vi "find_optimal_control_parameters.vi"() -> ()   [LabVIEW 2017]
uses:
  <vilib>/DAQmx/write.llb/DAQmx Write (Analog 1D Wfm NChan NSamp).vi
  <vilib>/DAQmx/create/channels.llb/DAQmx Create Channel (AO-Voltage-Basic).vi
  <vilib>/DAQmx/configure/timing.llb/DAQmx Timing (Sample Clock).vi
  <vilib>/DAQmx/miscellaneous.llb/DAQmx Fill In Error Info.vi
panel:
  in  "Camera delay (s)":dbl=0.5
  in  "Camera start phase":dbl=63.0
  in  "Exposure Time":dbl=0.00199
  in  "Camera Region":T1={"Horizontal Offset"=1020, "Vertical Offset"=820, "Horizontal Size"=580, "Vertical Size"=404}
  out "XY Graph":cluster{"Array":dbl[], "Array":dbl[]}(graph)
  in  "Stop":bool
  out "error out":errorcluster
  in  "Save data path":path=path "D:/"
  in  "Project name":string="syn data"
  in  "Number of Samples":i32=400000
  in  "Sample Rate":dbl=400000.0
  in  "Sample Clock Source":tag="OnboardClock"
  in  "Max Voltage":dbl=5.0
  in  "Min Voltage":dbl=-1.0
  in  "Physical Channel(s)":tag="PXI1Slot3_2/ao29, PXI1Slot3_2/ao31, PXI1Slot3_2/ao3"
  in  "Tab Control":T2(tab)
  in  "Frequency":dbl=50.0
  in  "Vgalvo phase Max":dbl=123.0
  in  "Vgalvo phase Min":dbl=113.0
  out "Vgalvo phase":dbl
  in  "Vgalvo offset":dbl
  in  "Vgalvo amplitude":dbl=0.068
  in  "Iteration times":i32=10
  in  "Vetl phase":dbl
  in  "Vetl amplitude":dbl=0.8
  in  "Vetl offset":dbl=2.0
  out "Vgalvo offset 2":dbl
  in  "Vgalvo offset Max 2":dbl=0.01
  in  "Vgalvo offset Min 2":dbl=-0.01
  in  "Iteration times 2":i32=10
  in  "Vgalvo phase 2":dbl=118.0
  in  "Vgalvo amplitude 2":dbl=0.068
  in  "Vetl phase 2":dbl
  in  "Vetl amplitude 2":dbl=0.8
  in  "Vetl offset 2":dbl=2.0
  in  "Frequency 2":dbl=50.0
  out "Vgalvo amp 3":dbl
  in  "Vgalvo amp Max 3":dbl=0.07
  in  "Vgalvo amp Min 3":dbl=0.066
  in  "Iteration times 3":i32=10
  in  "Vgalvo phase 3":dbl=118.0
  in  "Vgalvo offset 3":dbl
  in  "Vetl phase 3":dbl
  in  "Vetl amplitude 3":dbl=0.8
  in  "Vetl offset 3":dbl=2.0
  in  "Frequency 3":dbl=50.0
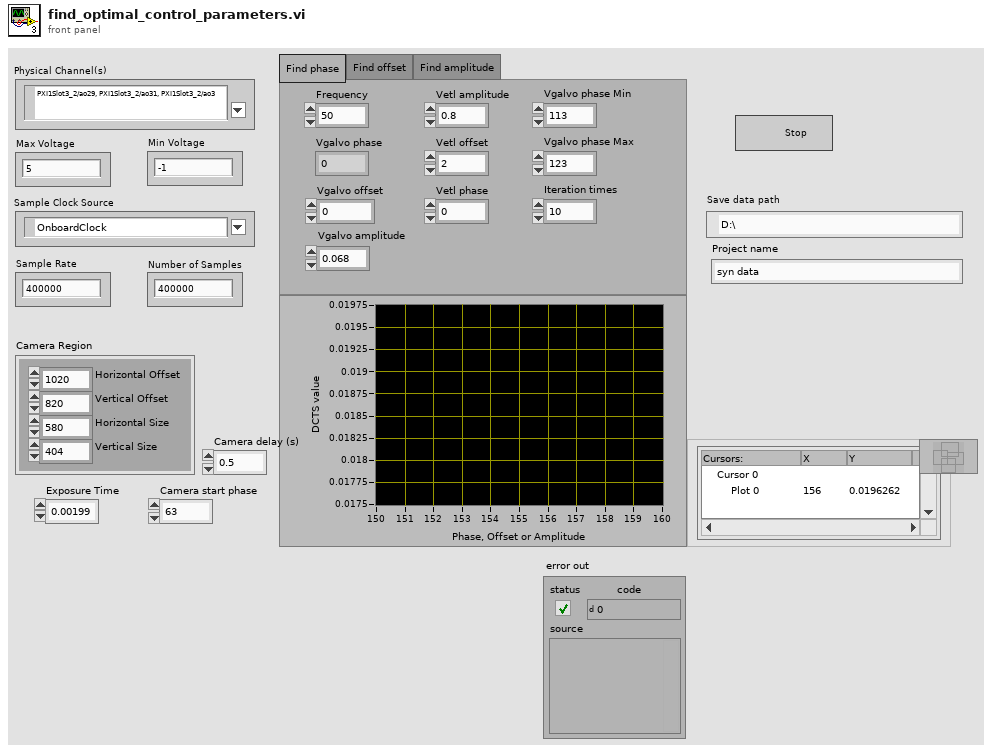
[diagram p1: front panel]
types:
  T1 = cluster{"Horizontal Offset":i32, "Vertical Offset":i32, "Horizontal Size":i32, "Vertical Size":i32}
  T2 = enum32{"Find phase", "Find offset", "Find amplitude"}
  T3 = enum16{"open", "replace", "create", "open or create", "replace or create", "replace or create with confirmation"}
  T4 = cluster{"frequency":dbl, "amplitude":dbl, "offset":dbl, "phase":dbl}
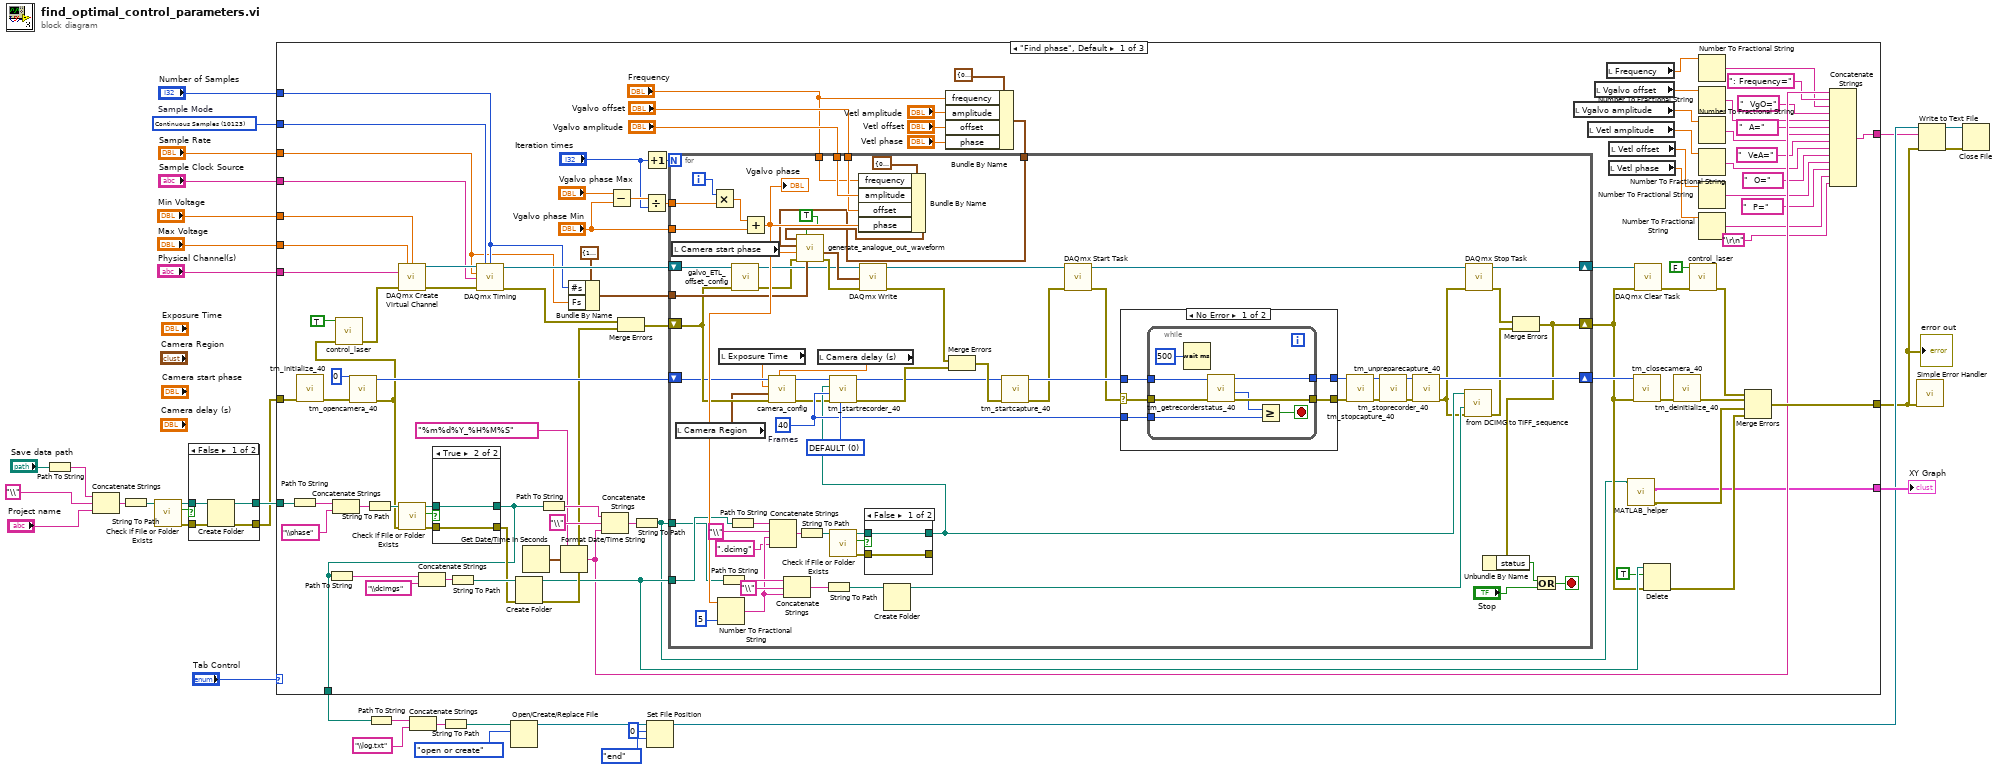
[diagram p0: block diagram]
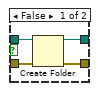
[diagram p3: hidden frame]
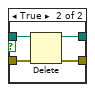
[diagram p5: hidden frame]
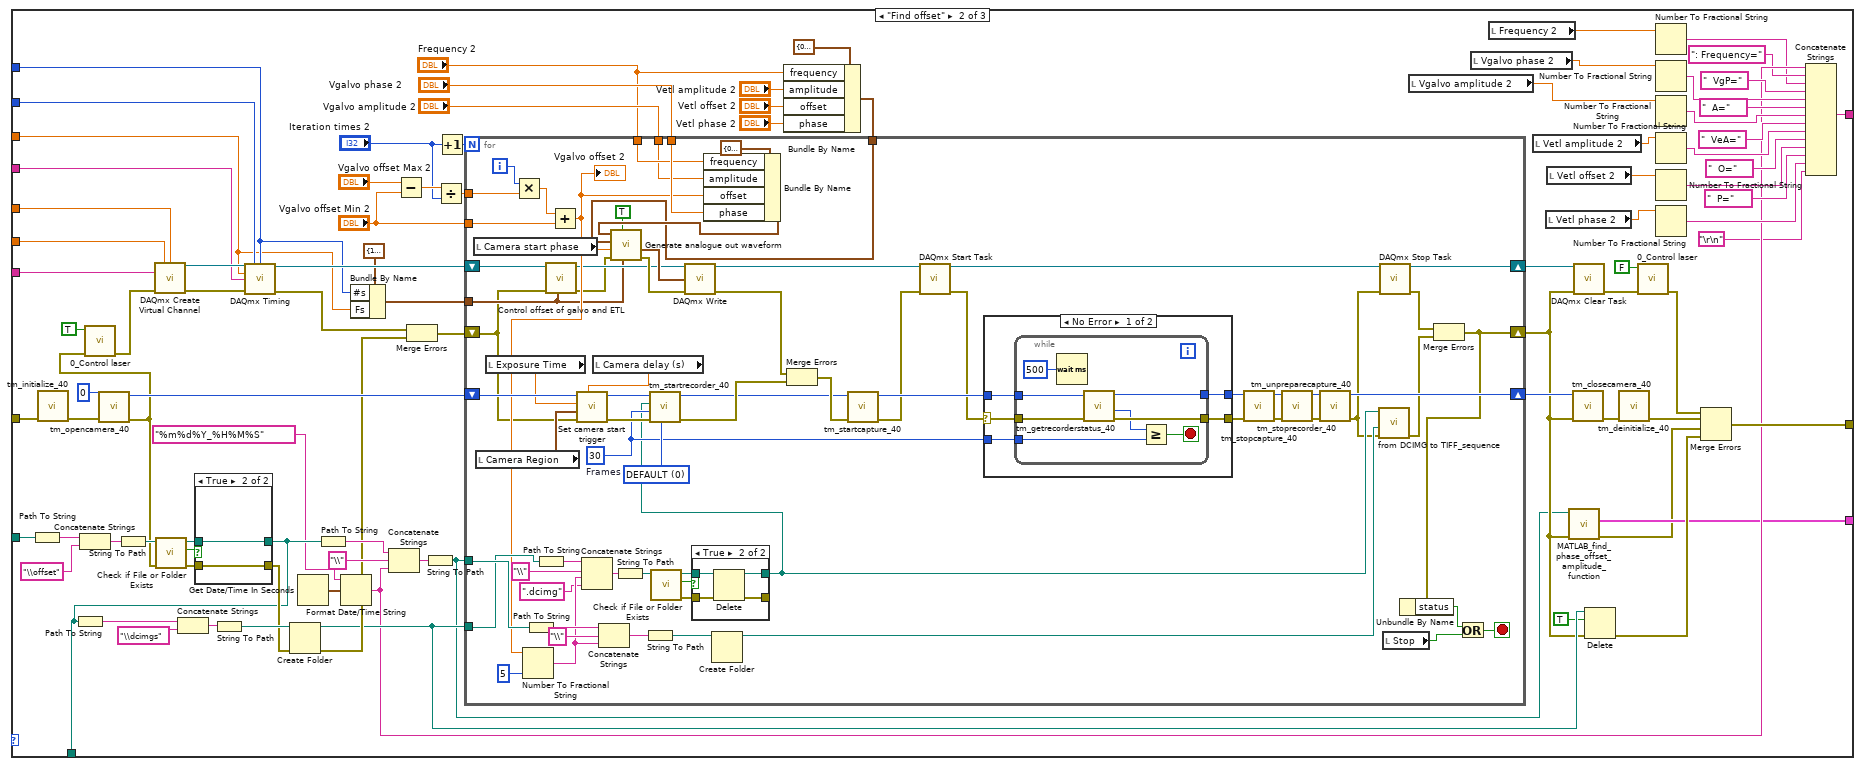
[diagram p6: hidden frame]
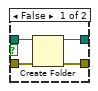
[diagram p7: hidden frame]
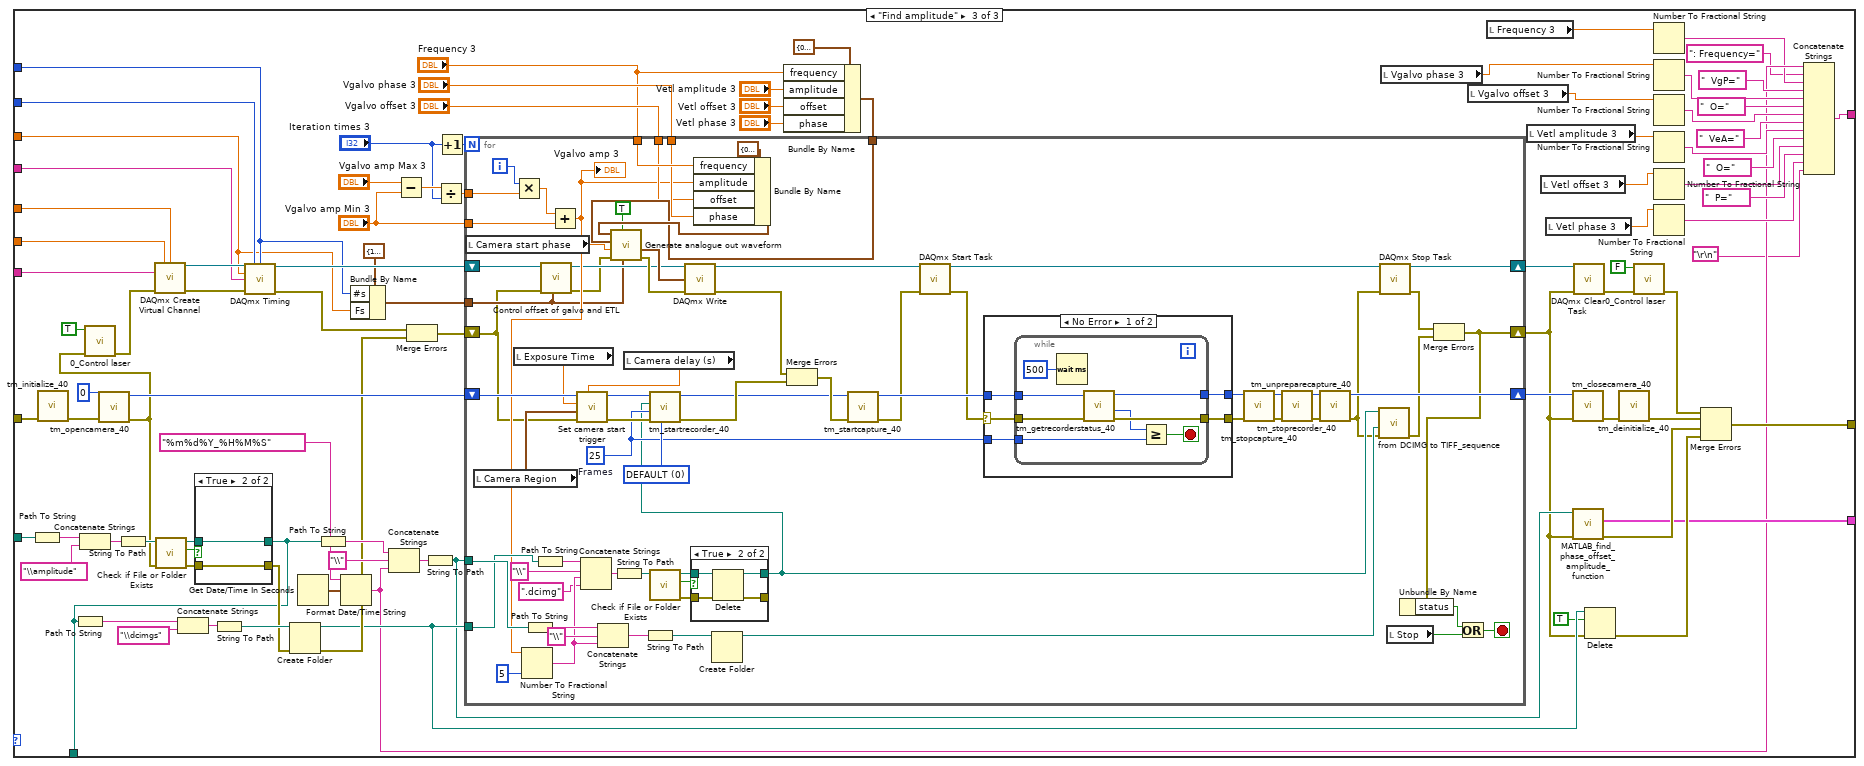
[diagram p10: hidden frame]
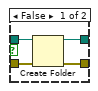
[diagram p11: hidden frame]
diagram:
  w23 = 10123 items=["Finite Samples"=10178, "Continuous Samples"=10123, "Hardware Timed Single Point"=12522]  # Sample Mode
  n1 = Path To String(path="Save data path") -> (string=w28:string)
  n2 = Concatenate Strings(w28, "\\", "Project name") -> (w27:string)
  n3 = String To Path(string=w27) -> (path=w33:path)
  n4 = call <vilib>:"Check if File or Folder Exists.vi"("path"=w33) -> ("error out"=w32:errorcluster, "file or folder exists?"=w31:bool, "dup path"=w30:path)  [unwired: 8 in]
  n5 = case shown="False" w31 {
    tunnel: w30 -> [w38 w39]
    tunnel: w32 -> [w37 w40]
    tunnel: [w36 w40] -> w1
    tunnel: [w35 w39] -> w26
    frame False {
      n6 = Create Folder(path (use dialog)=w38, error in=w37) -> (created path=w35:path, error out=w36:errorcluster)  [unwired: 1 in, 1 out]
    }
    frame True {
    }
  }
  n7 = case shown="\"Find phase\", Default" "Tab Control" {
    tunnel: w26 -> [w128 w264 w448]
    tunnel: w1 -> [w108 w263 w449]
    tunnel: w23 -> [w90 w270 w455]
    tunnel: "Number of Samples" -> [w84 w271 w456]
    tunnel: "Sample Rate" -> [w83 w269 w454]
    tunnel: "Sample Clock Source" -> [w89 w268 w453]
    tunnel: "Min Voltage" -> [w88 w267 w452]
    tunnel: "Max Voltage" -> [w87 w266 w451]
    tunnel: "Physical Channel(s)" -> [w86 w265 w450]
    tunnel: [w73 w262 w446] -> w3
    tunnel: [w44 w238 w447] -> w16
    tunnel: [w71 w250 w434] -> w12
    tunnel: [w53 w251 w435] -> w5
    frame "Find phase", Default {
      n8 = Path To String(path=w128) -> (string=w127:string)
      n9 = call <userlib>:"tm_initialize_40.vi"("error in (no error)"=w108) -> ("error out"=w123:errorcluster)  [unwired: 7 in, 3 out]
      n10 = Concatenate Strings(w127, "\\phase") -> (w125:string)
      n11 = call <userlib>:"tm_opencamera_40.vi"("error in (no error)"=w123, "Camera Index"=u32 0) -> ("error out"=w48:errorcluster, "Handle out"=w117:u32)  [unwired: 7 in, 1 out]
      n12 = call "control_laser.vi"("error in (no error)"=w48, "Laser On/Off"=TRUE ("Layser On/Off")) -> ("error out"=w49:errorcluster)  [unwired: 9 in]
      n13 = String To Path(string=w125) -> (path=w124:path)
      n14 = call-poly <vilib>:"DAQmx Create Virtual Channel.vi"("maximum value"=w87, "minimum value"=w88, "physical channels"=w86, "error in"=w49) -> ("task out"=w110:refnum<k21>, "error out"=w109:errorcluster)  [unwired: 10 in]
      n15 = call <vilib>:"Check if File or Folder Exists.vi"("error in (no error)"=w48, "path"=w124) -> ("error out"=w131:errorcluster, "file or folder exists?"=w130:bool, "dup path"=w129:path)  [unwired: 7 in]
      n16 = case shown="True" w130 {
        tunnel: w129 -> [w135 w136]
        tunnel: w131 -> [w134 w137]
        tunnel: [w133 w137] -> w93
        tunnel: [w132 w136] -> w71
        frame False {
          n17 = Create Folder(path (use dialog)=w135, error in=w134) -> (created path=w132:path, error out=w133:errorcluster)  [unwired: 1 in, 1 out]
        }
        frame True {
        }
      }
      n18 = Path To String(path=w71) -> (string=w118:string)
      n19 = Concatenate Strings(w118, "\\dcimgs") -> (w120:string)
      n20 = String To Path(string=w120) -> (path=w119:path)
      n21 = call-poly <vilib>:"DAQmx Timing.vi"("task/channels in"=w110, "sample mode"=w90, "samples per channel"=w84, "rate"=w83, "source"=w89, "error in"=w109) -> ("task out"=w105:refnum<k21>, "error out"=w94:errorcluster)  [unwired: 8 in]
      n22 = Create Folder(path (use dialog)=w119, error in=w93) -> (created path=w78:path, error out=w92:errorcluster)  [unwired: 1 in, 1 out]
      n23 = Get Date/Time In Seconds() -> (seconds since 1Jan1904=w104:timestamp)
      n24 = Path To String(path=w71) -> (string=w101:string)
      n25 = Format Date/Time String(time format string (%c)="%m%d%Y_%H%M%S", seconds (now)=w104) -> (date/time string=w64:string)  [unwired: 1 in]
      n26 = Bundle By Name(cluster=cluster{"Fs":dbl, "#s":dbl} {"Fs"=1000.0, "#s"=1000.0} ("sampling info"), "#s"=w84, "Fs"=w83) -> (w82:cluster{"Fs":dbl, "#s":dbl})
      n27 = Concatenate Strings(w101, "\\", w64) -> (w102:string)
      n28 = Subtract(x="Vgalvo phase Max", y="Vgalvo phase Min") -> (x-y=w115:dbl)
      n29 = Merge Errors(w94, w92) -> (w91:errorcluster)
      n30 = String To Path(string=w102) -> (path=w45:path)
      n31 = Divide(x=w115, y="Iteration times") -> (x/y=w112:dbl)
      n32 = Increment(x="Iteration times") -> (x+1=w113:i32)
      n33 = Bundle By Name(cluster=T4 {"frequency"=0.0, "amplitude"=0.0, "offset"=0.0, "phase"=0.0}, "frequency"="Frequency", "amplitude"="Vetl amplitude", "offset"="Vetl offset", "phase"="Vetl phase") -> (w95:T4)
      n34 = for {
        N: w113 -> [_]
        tunnel: w78 -> [w157]
        tunnel: w112 -> [w207]
        tunnel: "Vgalvo phase Min" -> [w204]
        tunnel: "Vgalvo offset" -> [w177]
        tunnel: "Vgalvo amplitude" -> [w178]
        tunnel: w45 -> [w156]
        tunnel: "Frequency" -> [w175]
        tunnel: w95 -> [w153]
        shift-right: [w164] -> w76
        shift-left: w91 -> [w144]
        shift-right: [w169] -> w80
        shift-left: w117 -> [w141]
        shift-right: [w168] -> w81
        shift-left: w105 -> [w147]
        tunnel: w82 -> [w148]
        i -> [w206]
        stop <- w163 stop-if-true
        w200 = 0 items=["DEFAULT", "NO BUFFERING"] ("Buffering Mode")
        w183 = 40  # Frames
        n35 = local read "Camera start phase"() -> (w152:dbl)
        n36 = local read "Camera Region"() -> (w140:T1)
        n37 = Multiply(x=w206, y=w207) -> (x*y=w205:dbl)
        n38 = local read "Exposure Time"() -> (w139:dbl)
        n39 = Path To String(path=w156) -> (string=w191:string)
        n40 = Path To String(path=w157) -> (string=w199:string)
        n41 = call "galvo_ETL_offset_config.vi"("error in (no error)"=w144, "task/channels in"=w147) -> ("error out"=w145:errorcluster, "task out"=w146:refnum<k21>)  [unwired: 8 in]
        n42 = Add(x=w205, y=w204) -> (x+y=w176:dbl)
        "Vgalvo phase" <- w176
        n43 = Number To Fractional String(number=w176, precision (6)=5) -> (F-format string=w159:string)  [unwired: 2 in]
        n44 = Concatenate Strings(w199, "\\", w159, ".dcimg") -> (w198:string)
        n45 = Concatenate Strings(w191, "\\", w159) -> (w192:string)
        n46 = String To Path(string=w198) -> (path=w194:path)
        n47 = local read "Camera delay (s)"() -> (w138:dbl)
        n48 = call "camera_config.vi"("Cam Delay"=w138, "error in (no error)"=w144, "Sub Region"=w140, "Exposure Time(s)"=w139, "Handle in"=w141) -> ("error out"=w143:errorcluster, "Handle out"=w142:u32)  [unwired: 5 in]
        n49 = String To Path(string=w192) -> (path=w193:path)
        n50 = call <vilib>:"Check if File or Folder Exists.vi"("path"=w194) -> ("error out"=w196:errorcluster, "file or folder exists?"=w195:bool, "dup path"=w197:path)  [unwired: 8 in]
        n51 = Bundle By Name(cluster=T4 {"frequency"=0.0, "amplitude"=0.0, "offset"=0.0, "phase"=0.0}, "frequency"=w175, "amplitude"=w178, "offset"=w177, "phase"=w176) -> (w154:T4)
        n52 = call "generate_analogue_out_waveform.vi"("sampling info"=w148, "Reset signal"=TRUE, "error in (no error)"=w145, "Camera start trigger phase"=w152, "Vetl sine"=w153, "Vgalvo sine"=w154) -> ("error out"=w149:errorcluster, "Waveform Graph"=w151:waveform(dbl)[])  [unwired: 4 in]
        n53 = call-poly <vilib>:"DAQmx Write.vi"("task/channels in"=w146, "data"=w151, "error in"=w149) -> ("task out"=w180:refnum<k21>, "error out"=w179:errorcluster)  [unwired: 10 in, 1 out]
        n54 = case shown="False" w195 {
          tunnel: w196 -> [w224 w228]
          tunnel: [w224 w227] -> _
          tunnel: w197 -> [w223 w226]
          tunnel: [w223 w225] -> w173
          frame False {
          }
          frame True {
            n55 = Delete(path (use dialog)=w226, error in=w228) -> (deleted path=w225:path, error out=w227:errorcluster)  [unwired: 3 in, 1 out]
          }
        }
        n56 = call <userlib>:"tm_startrecorder_40.vi"("Buffering Mode"=w200, "error in (no error)"=w143, "frames"=w183, "File"=w173, "Handle in"=w142) -> ("error out"=w203:errorcluster, "Handle out"=w201:u32)  [unwired: 5 in]
        n57 = Create Folder(path (use dialog)=w193) -> (created path=w172:path)  [unwired: 2 in, 2 out]
        n58 = Merge Errors(w179, w203) -> (w202:errorcluster)
        n59 = call <userlib>:"tm_startcapture_40.vi"("error in (no error)"=w202, "Handle in"=w201) -> ("error out"=w182:errorcluster, "Handle out"=w184:u32)  [unwired: 8 in]
        n60 = call <vilib>:"DAQmx Start Task.vi"("task/channels in"=w180, "error in"=w182) -> ("task out"=w171:refnum<k21>, "error out"=w181:errorcluster)  [unwired: 12 in]
        n61 = case shown="No Error" w181 {
          selector: w181 -> [w212 w222]
          tunnel: [w210 w221] -> w188
          tunnel: [w209 w222] -> w187
          tunnel: w183 -> [w211 _]
          tunnel: w184 -> [w208 w221]
          frame No Error {
            n62 = while {
              tunnel: w212 -> [w218]
              tunnel: [w217] -> w209
              tunnel: [w219] -> w210
              tunnel: w211 -> [w220]
              tunnel: w208 -> [w213]
              stop <- w214 stop-if-true
              n63 = Wait (ms)(milliseconds to wait=u32 500) -> ()  [unwired: 1 out]
              n64 = call <userlib>:"tm_getrecorderstatus_40.vi"("error in (no error)"=w218, "Handle"=w213) -> ("error out"=w217:errorcluster, "Count"=w216:i32, "Handle"=w219:u32)  [unwired: 6 in, 1 out]
              n65 = Greater Or Equal?(x=w216, y=w220) -> (x >= y?=w214:bool)
            }
          }
          frame Error {
          }
        }
        n66 = call <userlib>:"tm_stopcapture_40.vi"("error in (no error)"=w187, "Handle in"=w188) -> ("error out"=w185:errorcluster, "Handle out"=w186:u32)  [unwired: 8 in]
        n67 = call <userlib>:"tm_stoprecorder_40.vi"("error in (no error)"=w185, "Handle in"=w186) -> ("error out"=w189:errorcluster, "Handle out"=w190:u32)  [unwired: 8 in]
        n68 = call <userlib>:"tm_unpreparecapture_40.vi"("error in (no error)"=w189, "Handle in"=w190) -> ("error out"=w166:errorcluster, "Handle out"=w169:u32)  [unwired: 8 in]
        n69 = call "from DCIMG to TIFF_sequence.vi"("error in (no error)"=w166, "Where to Store"=w172, "DCIMG Path"=w173) -> ("Error Out"=w165:errorcluster)  [unwired: 7 in, 1 out]
        n70 = call <vilib>:"DAQmx Stop Task.vi"("task/channels in"=w171, "error in"=w166) -> ("task out"=w168:refnum<k21>, "error out"=w167:errorcluster)  [unwired: 12 in]
        n71 = Merge Errors(w167, w165) -> (w164:errorcluster)
        n72 = Unbundle By Name(w164) -> ("status"=w170:bool)
        n73 = Or(x=w170, y="Stop") -> (x .or. y?=w163:bool)
      }
      n74 = local read "Vgalvo amplitude"() -> (w68:dbl)
      n75 = local read "Vetl amplitude"() -> (w67:dbl)
      n76 = local read "Vgalvo offset"() -> (w69:dbl)
      n77 = local read "Frequency"() -> (w70:dbl)
      n78 = local read "Vetl phase"() -> (w65:dbl)
      n79 = local read "Vetl offset"() -> (w66:dbl)
      n80 = call "MATLAB_helper.vi"("Path"=w45) -> ("error out"=w46:errorcluster, "XY Graph"=w44:cluster{"Array":dbl[], "Array":dbl[]})  [unwired: 8 in, 1 out]
      n81 = call <userlib>:"tm_closecamera_40.vi"("error in (no error)"=w76, "Handle in"=w80) -> ("error out"=w79:errorcluster)  [unwired: 9 in]
      n82 = call <vilib>:"DAQmx Clear Task.vi"("task in"=w81, "error in"=w76) -> ("error out"=w43:errorcluster)  [unwired: 13 in]
      n83 = Delete(path (use dialog)=w78, entire hierarchy (F)=TRUE, error in=w76) -> (error out=w74:errorcluster)  [unwired: 2 in, 2 out]
      n84 = call <userlib>:"tm_deinitialize_40.vi"("error in (no error)"=w79) -> ("error out"=w75:errorcluster)  [unwired: 10 in]
      n85 = call "control_laser.vi"("error in (no error)"=w43, "Laser On/Off"=FALSE ("Layser On/Off")) -> ("error out"=w42:errorcluster)  [unwired: 9 in]
      n86 = Number To Fractional String(number=w70) -> (F-format string=w50:string)  [unwired: 3 in]
      n87 = Number To Fractional String(number=w69) -> (F-format string=w62:string)  [unwired: 3 in]
      n88 = Number To Fractional String(number=w68) -> (F-format string=w60:string)  [unwired: 3 in]
      n89 = Number To Fractional String(number=w67) -> (F-format string=w58:string)  [unwired: 3 in]
      n90 = Number To Fractional String(number=w66) -> (F-format string=w56:string)  [unwired: 3 in]
      n91 = Number To Fractional String(number=w65) -> (F-format string=w54:string)  [unwired: 3 in]
      n92 = Merge Errors(w42, w75, w46, w74) -> (w73:errorcluster)
      n93 = Concatenate Strings(w64, ": Frequency=", w50, "  VgO=", w62, "  A=", w60, "  VeA=", w58, "  O=", w56, "  P=", w54, "\r\n") -> (w53:string)
    }
    frame "Find offset" {
      n94 = Path To String(path=w264) -> (string=w316:string)
      n95 = call <userlib>:"tm_initialize_40.vi"("error in (no error)"=w263) -> ("error out"=w312:errorcluster)  [unwired: 7 in, 3 out]
      n96 = Concatenate Strings(w316, "\\offset") -> (w314:string)
      n97 = call <userlib>:"tm_opencamera_40.vi"("error in (no error)"=w312, "Camera Index"=u32 0) -> ("error out"=w233:errorcluster, "Handle out"=w306:u32)  [unwired: 7 in, 1 out]
      n98 = call "0_Control laser.vi"("error in (no error)"=w233, "Laser On/Off"=TRUE ("Layser On/Off")) -> ("error out"=w234:errorcluster)  [unwired: 9 in]
      n99 = String To Path(string=w314) -> (path=w313:path)
      n100 = call-poly <vilib>:"DAQmx Create Virtual Channel.vi"("maximum value"=w266, "minimum value"=w267, "physical channels"=w265, "error in"=w234) -> ("task out"=w299:refnum<k21>, "error out"=w298:errorcluster)  [unwired: 10 in]
      n101 = call <vilib>:"Check if File or Folder Exists.vi"("error in (no error)"=w233, "path"=w313) -> ("error out"=w319:errorcluster, "file or folder exists?"=w318:bool, "dup path"=w317:path)  [unwired: 7 in]
      n102 = case shown="True" w318 {
        tunnel: w317 -> [w323 w324]
        tunnel: w319 -> [w322 w325]
        tunnel: [w321 w325] -> w283
        tunnel: [w320 w324] -> w250
        frame False {
          n103 = Create Folder(path (use dialog)=w323, error in=w322) -> (created path=w320:path, error out=w321:errorcluster)  [unwired: 1 in, 1 out]
        }
        frame True {
        }
      }
      n104 = Path To String(path=w250) -> (string=w307:string)
      n105 = Concatenate Strings(w307, "\\dcimgs") -> (w309:string)
      n106 = String To Path(string=w309) -> (path=w308:path)
      n107 = call-poly <vilib>:"DAQmx Timing.vi"("task/channels in"=w299, "sample mode"=w270, "samples per channel"=w271, "rate"=w269, "source"=w268, "error in"=w298) -> ("task out"=w295:refnum<k21>, "error out"=w284:errorcluster)  [unwired: 8 in]
      n108 = Create Folder(path (use dialog)=w308, error in=w283) -> (created path=w275:path, error out=w282:errorcluster)  [unwired: 1 in, 1 out]
      n109 = Get Date/Time In Seconds() -> (seconds since 1Jan1904=w294:timestamp)
      n110 = Path To String(path=w250) -> (string=w291:string)
      n111 = Format Date/Time String(time format string (%c)="%m%d%Y_%H%M%S", seconds (now)=w294) -> (date/time string=w249:string)  [unwired: 1 in]
      n112 = Bundle By Name(cluster=cluster{"Fs":dbl, "#s":dbl} {"Fs"=1000.0, "#s"=1000.0} ("sampling info"), "#s"=w271, "Fs"=w269) -> (w279:cluster{"Fs":dbl, "#s":dbl})
      n113 = Concatenate Strings(w291, "\\", w249) -> (w292:string)
      n114 = Subtract(x="Vgalvo offset Max 2", y="Vgalvo offset Min 2") -> (x-y=w304:dbl)
      n115 = Merge Errors(w284, w282) -> (w281:errorcluster)
      n116 = String To Path(string=w292) -> (path=w235:path)
      n117 = Divide(x=w304, y="Iteration times 2") -> (x/y=w301:dbl)
      n118 = Increment(x="Iteration times 2") -> (x+1=w302:i32)
      n119 = Bundle By Name(cluster=T4 {"frequency"=0.0, "amplitude"=0.0, "offset"=0.0, "phase"=0.0}, "frequency"="Frequency 2", "amplitude"="Vetl amplitude 2", "offset"="Vetl offset 2", "phase"="Vetl phase 2") -> (w285:T4)
      n120 = for {
        N: w302 -> [_]
        tunnel: w275 -> [w336]
        tunnel: w301 -> [w392]
        tunnel: "Vgalvo offset Min 2" -> [w389]
        tunnel: "Vgalvo phase 2" -> [w350]
        tunnel: "Vgalvo amplitude 2" -> [w348]
        tunnel: w235 -> [w337]
        tunnel: "Frequency 2" -> [w349]
        tunnel: w285 -> [w363]
        shift-right: [w352] -> w236
        shift-left: w281 -> [w328]
        shift-right: [w357] -> w277
        shift-left: w306 -> [w395]
        shift-right: [w356] -> w278
        shift-left: w295 -> [w331]
        tunnel: w279 -> [w329]
        i -> [w391]
        stop <- w351 stop-if-true
        w385 = 0 items=["DEFAULT", "NO BUFFERING"] ("Buffering Mode")
        w372 = 30  # Frames
        n121 = local read "Camera start phase"() -> (w344:dbl)
        n122 = local read "Camera Region"() -> (w346:T1)
        n123 = local read "Exposure Time"() -> (w345:dbl)
        n124 = Multiply(x=w391, y=w392) -> (x*y=w390:dbl)
        n125 = Path To String(path=w337) -> (string=w342:string)
        n126 = Path To String(path=w336) -> (string=w343:string)
        n127 = call "Control offset of galvo and ETL.vi"("sampling info"=w329, "error in (no error)"=w328, "task/channels in"=w331) -> ("error out"=w327:errorcluster, "task out"=w330:refnum<k21>)  [unwired: 7 in]
        n128 = Add(x=w390, y=w389) -> (x+y=w334:dbl)
        "Vgalvo offset 2" <- w334
        n129 = Number To Fractional String(number=w334, precision (6)=5) -> (F-format string=w339:string)  [unwired: 2 in]
        n130 = Concatenate Strings(w343, "\\", w339, ".dcimg") -> (w332:string)
        n131 = local read "Camera delay (s)"() -> (w326:dbl)
        n132 = call "Set camera start trigger.vi"("Cam Delay"=w326, "error in (no error)"=w328, "Sub Region"=w346, "Exposure Time(s)"=w345, "Handle in"=w395) -> ("error out"=w393:errorcluster, "Handle out"=w394:u32)  [unwired: 5 in]
        n133 = Concatenate Strings(w342, "\\", w339) -> (w335:string)
        n134 = String To Path(string=w332) -> (path=w381:path)
        n135 = String To Path(string=w335) -> (path=w380:path)
        n136 = call <vilib>:"Check if File or Folder Exists.vi"("path"=w381) -> ("error out"=w383:errorcluster, "file or folder exists?"=w382:bool, "dup path"=w384:path)  [unwired: 8 in]
        n137 = case shown="True" w382 {
          tunnel: w383 -> [w412 w416]
          tunnel: [w412 w415] -> _
          tunnel: w384 -> [w411 w414]
          tunnel: [w411 w413] -> w361
          frame False {
          }
          frame True {
            n138 = Delete(path (use dialog)=w414, error in=w416) -> (deleted path=w413:path, error out=w415:errorcluster)  [unwired: 3 in, 1 out]
          }
        }
        n139 = call <userlib>:"tm_startrecorder_40.vi"("Buffering Mode"=w385, "error in (no error)"=w393, "frames"=w372, "File"=w361, "Handle in"=w394) -> ("error out"=w388:errorcluster, "Handle out"=w386:u32)  [unwired: 5 in]
        n140 = Bundle By Name(cluster=T4 {"frequency"=0.0, "amplitude"=0.0, "offset"=0.0, "phase"=0.0}, "frequency"=w349, "amplitude"=w348, "offset"=w334, "phase"=w350) -> (w364:T4)
        n141 = call "Generate analogue out waveform.vi"("sampling info"=w329, "Reset signal"=TRUE, "error in (no error)"=w327, "Camera start trigger phase"=w344, "Vetl sine"=w363, "Vgalvo sine"=w364) -> ("error out"=w366:errorcluster, "Waveform Graph"=w365:waveform(dbl)[])  [unwired: 4 in]
        n142 = call-poly <vilib>:"DAQmx Write.vi"("task/channels in"=w330, "data"=w365, "error in"=w366) -> ("task out"=w369:refnum<k21>, "error out"=w368:errorcluster)  [unwired: 10 in, 1 out]
        n143 = Create Folder(path (use dialog)=w380) -> (created path=w360:path)  [unwired: 2 in, 2 out]
        n144 = Merge Errors(w368, w388) -> (w387:errorcluster)
        n145 = call <userlib>:"tm_startcapture_40.vi"("error in (no error)"=w387, "Handle in"=w386) -> ("error out"=w371:errorcluster, "Handle out"=w373:u32)  [unwired: 8 in]
        n146 = call <vilib>:"DAQmx Start Task.vi"("task/channels in"=w369, "error in"=w371) -> ("task out"=w359:refnum<k21>, "error out"=w370:errorcluster)  [unwired: 12 in]
        n147 = case shown="No Error" w370 {
          selector: w370 -> [w400 w410]
          tunnel: [w398 w409] -> w377
          tunnel: [w397 w410] -> w376
          tunnel: w372 -> [w399 _]
          tunnel: w373 -> [w396 w409]
          frame No Error {
            n148 = while {
              tunnel: w400 -> [w406]
              tunnel: [w405] -> w397
              tunnel: [w407] -> w398
              tunnel: w399 -> [w408]
              tunnel: w396 -> [w401]
              stop <- w402 stop-if-true
              n149 = Wait (ms)(milliseconds to wait=u32 500) -> ()  [unwired: 1 out]
              n150 = call <userlib>:"tm_getrecorderstatus_40.vi"("error in (no error)"=w406, "Handle"=w401) -> ("error out"=w405:errorcluster, "Count"=w404:i32, "Handle"=w407:u32)  [unwired: 6 in, 1 out]
              n151 = Greater Or Equal?(x=w404, y=w408) -> (x >= y?=w402:bool)
            }
          }
          frame Error {
          }
        }
        n152 = call <userlib>:"tm_stopcapture_40.vi"("error in (no error)"=w376, "Handle in"=w377) -> ("error out"=w374:errorcluster, "Handle out"=w375:u32)  [unwired: 8 in]
        n153 = call <userlib>:"tm_stoprecorder_40.vi"("error in (no error)"=w374, "Handle in"=w375) -> ("error out"=w378:errorcluster, "Handle out"=w379:u32)  [unwired: 8 in]
        n154 = call <userlib>:"tm_unpreparecapture_40.vi"("error in (no error)"=w378, "Handle in"=w379) -> ("error out"=w354:errorcluster, "Handle out"=w357:u32)  [unwired: 8 in]
        n155 = call "from DCIMG to TIFF_sequence.vi"("error in (no error)"=w354, "Where to Store"=w360, "DCIMG Path"=w361) -> ("Error Out"=w353:errorcluster)  [unwired: 7 in, 1 out]
        n156 = call <vilib>:"DAQmx Stop Task.vi"("task/channels in"=w359, "error in"=w354) -> ("task out"=w356:refnum<k21>, "error out"=w355:errorcluster)  [unwired: 12 in]
        n157 = local read "Stop"() -> (w347:bool)
        n158 = Merge Errors(w355, w353) -> (w352:errorcluster)
        n159 = Unbundle By Name(w352) -> ("status"=w358:bool)
        n160 = Or(x=w358, y=w347) -> (x .or. y?=w351:bool)
      }
      n161 = local read "Vgalvo amplitude 2"() -> (w246:dbl)
      n162 = local read "Vgalvo phase 2"() -> (w247:dbl)
      n163 = local read "Frequency 2"() -> (w248:dbl)
      n164 = local read "Vetl amplitude 2"() -> (w245:dbl)
      n165 = local read "Vetl phase 2"() -> (w243:dbl)
      n166 = local read "Vetl offset 2"() -> (w244:dbl)
      n167 = call "MATLAB_find_phase_offset_amplitude_function.vi"("error in (no error)"=w236, "Path"=w235) -> ("error out"=w237:errorcluster, "XY Graph"=w238:cluster{"Array":dbl[], "Array":dbl[]})  [unwired: 7 in, 1 out]
      n168 = call <userlib>:"tm_closecamera_40.vi"("error in (no error)"=w236, "Handle in"=w277) -> ("error out"=w276:errorcluster)  [unwired: 9 in]
      n169 = call <vilib>:"DAQmx Clear Task.vi"("task in"=w278, "error in"=w236) -> ("error out"=w230:errorcluster)  [unwired: 13 in]
      n170 = Delete(path (use dialog)=w275, entire hierarchy (F)=TRUE, error in=w236) -> (error out=w272:errorcluster)  [unwired: 2 in, 2 out]
      n171 = call <userlib>:"tm_deinitialize_40.vi"("error in (no error)"=w276) -> ("error out"=w273:errorcluster)  [unwired: 10 in]
      n172 = call "0_Control laser.vi"("error in (no error)"=w230, "Laser On/Off"=FALSE ("Layser On/Off")) -> ("error out"=w231:errorcluster)  [unwired: 9 in]
      n173 = Number To Fractional String(number=w248) -> (F-format string=w240:string)  [unwired: 3 in]
      n174 = Number To Fractional String(number=w247) -> (F-format string=w260:string)  [unwired: 3 in]
      n175 = Number To Fractional String(number=w246) -> (F-format string=w258:string)  [unwired: 3 in]
      n176 = Number To Fractional String(number=w245) -> (F-format string=w256:string)  [unwired: 3 in]
      n177 = Number To Fractional String(number=w244) -> (F-format string=w254:string)  [unwired: 3 in]
      n178 = Number To Fractional String(number=w243) -> (F-format string=w252:string)  [unwired: 3 in]
      n179 = Merge Errors(w231, w273, w237, w272) -> (w262:errorcluster)
      n180 = Concatenate Strings(w249, ": Frequency=", w240, "  VgP=", w260, "  A=", w258, "  VeA=", w256, "  O=", w254, "  P=", w252, "\r\n") -> (w251:string)
    }
    frame "Find amplitude" {
      n181 = Path To String(path=w448) -> (string=w504:string)
      n182 = call <userlib>:"tm_initialize_40.vi"("error in (no error)"=w449) -> ("error out"=w500:errorcluster)  [unwired: 7 in, 3 out]
      n183 = Concatenate Strings(w504, "\\amplitude") -> (w502:string)
      n184 = call <userlib>:"tm_opencamera_40.vi"("error in (no error)"=w500, "Camera Index"=u32 0) -> ("error out"=w421:errorcluster, "Handle out"=w494:u32)  [unwired: 7 in, 1 out]
      n185 = call "0_Control laser.vi"("error in (no error)"=w421, "Laser On/Off"=TRUE ("Layser On/Off")) -> ("error out"=w422:errorcluster)  [unwired: 9 in]
      n186 = String To Path(string=w502) -> (path=w501:path)
      n187 = call-poly <vilib>:"DAQmx Create Virtual Channel.vi"("maximum value"=w451, "minimum value"=w452, "physical channels"=w450, "error in"=w422) -> ("task out"=w487:refnum<k21>, "error out"=w486:errorcluster)  [unwired: 10 in]
      n188 = call <vilib>:"Check if File or Folder Exists.vi"("error in (no error)"=w421, "path"=w501) -> ("error out"=w507:errorcluster, "file or folder exists?"=w506:bool, "dup path"=w505:path)  [unwired: 7 in]
      n189 = case shown="True" w506 {
        tunnel: w505 -> [w511 w512]
        tunnel: w507 -> [w510 w513]
        tunnel: [w509 w513] -> w471
        tunnel: [w508 w512] -> w434
        frame False {
          n190 = Create Folder(path (use dialog)=w511, error in=w510) -> (created path=w508:path, error out=w509:errorcluster)  [unwired: 1 in, 1 out]
        }
        frame True {
        }
      }
      n191 = Path To String(path=w434) -> (string=w495:string)
      n192 = Concatenate Strings(w495, "\\dcimgs") -> (w497:string)
      n193 = String To Path(string=w497) -> (path=w496:path)
      n194 = call-poly <vilib>:"DAQmx Timing.vi"("task/channels in"=w487, "sample mode"=w455, "samples per channel"=w456, "rate"=w454, "source"=w453, "error in"=w486) -> ("task out"=w483:refnum<k21>, "error out"=w472:errorcluster)  [unwired: 8 in]
      n195 = Create Folder(path (use dialog)=w496, error in=w471) -> (created path=w463:path, error out=w470:errorcluster)  [unwired: 1 in, 1 out]
      n196 = Get Date/Time In Seconds() -> (seconds since 1Jan1904=w482:timestamp)
      n197 = Path To String(path=w434) -> (string=w479:string)
      n198 = Format Date/Time String(time format string (%c)="%m%d%Y_%H%M%S", seconds (now)=w482) -> (date/time string=w433:string)  [unwired: 1 in]
      n199 = Bundle By Name(cluster=cluster{"Fs":dbl, "#s":dbl} {"Fs"=1000.0, "#s"=1000.0} ("sampling info"), "#s"=w456, "Fs"=w454) -> (w467:cluster{"Fs":dbl, "#s":dbl})
      n200 = Concatenate Strings(w479, "\\", w433) -> (w480:string)
      n201 = Subtract(x="Vgalvo amp Max 3", y="Vgalvo amp Min 3") -> (x-y=w492:dbl)
      n202 = Merge Errors(w472, w470) -> (w469:errorcluster)
      n203 = String To Path(string=w480) -> (path=w461:path)
      n204 = Divide(x=w492, y="Iteration times 3") -> (x/y=w489:dbl)
      n205 = Increment(x="Iteration times 3") -> (x+1=w490:i32)
      n206 = Bundle By Name(cluster=T4 {"frequency"=0.0, "amplitude"=0.0, "offset"=0.0, "phase"=0.0}, "frequency"="Frequency 3", "amplitude"="Vetl amplitude 3", "offset"="Vetl offset 3", "phase"="Vetl phase 3") -> (w473:T4)
      n207 = for {
        N: w490 -> [_]
        tunnel: w463 -> [w523]
        tunnel: w489 -> [w580]
        tunnel: "Vgalvo amp Min 3" -> [w577]
        tunnel: "Vgalvo phase 3" -> [w536]
        tunnel: "Vgalvo offset 3" -> [w535]
        tunnel: w461 -> [w524]
        tunnel: "Frequency 3" -> [w555]
        tunnel: w473 -> [w550]
        shift-right: [w539] -> w460
        shift-left: w469 -> [w515]
        shift-right: [w544] -> w465
        shift-left: w494 -> [w583]
        shift-right: [w543] -> w466
        shift-left: w483 -> [w519]
        tunnel: w467 -> [w517]
        i -> [w579]
        stop <- w538 stop-if-true
        w573 = 0 items=["DEFAULT", "NO BUFFERING"] ("Buffering Mode")
        w560 = 25  # Frames
        n208 = local read "Camera start phase"() -> (w532:dbl)
        n209 = local read "Camera Region"() -> (w534:T1)
        n210 = Multiply(x=w579, y=w580) -> (x*y=w578:dbl)
        n211 = local read "Exposure Time"() -> (w533:dbl)
        n212 = Path To String(path=w524) -> (string=w530:string)
        n213 = Path To String(path=w523) -> (string=w531:string)
        n214 = call "Control offset of galvo and ETL.vi"("sampling info"=w517, "error in (no error)"=w515, "task/channels in"=w519) -> ("error out"=w516:errorcluster, "task out"=w518:refnum<k21>)  [unwired: 7 in]
        n215 = Add(x=w578, y=w577) -> (x+y=w522:dbl)
        "Vgalvo amp 3" <- w522
        n216 = Number To Fractional String(number=w522, precision (6)=5) -> (F-format string=w527:string)  [unwired: 2 in]
        n217 = Concatenate Strings(w531, "\\", w527, ".dcimg") -> (w520:string)
        n218 = Concatenate Strings(w530, "\\", w527) -> (w521:string)
        n219 = String To Path(string=w520) -> (path=w569:path)
        n220 = local read "Camera delay (s)"() -> (w514:dbl)
        n221 = call "Set camera start trigger.vi"("Cam Delay"=w514, "error in (no error)"=w515, "Sub Region"=w534, "Exposure Time(s)"=w533, "Handle in"=w583) -> ("error out"=w581:errorcluster, "Handle out"=w582:u32)  [unwired: 5 in]
        n222 = String To Path(string=w521) -> (path=w568:path)
        n223 = call <vilib>:"Check if File or Folder Exists.vi"("path"=w569) -> ("error out"=w571:errorcluster, "file or folder exists?"=w570:bool, "dup path"=w572:path)  [unwired: 8 in]
        n224 = case shown="True" w570 {
          tunnel: w571 -> [w600 w604]
          tunnel: [w600 w603] -> _
          tunnel: w572 -> [w599 w602]
          tunnel: [w599 w601] -> w548
          frame False {
          }
          frame True {
            n225 = Delete(path (use dialog)=w602, error in=w604) -> (deleted path=w601:path, error out=w603:errorcluster)  [unwired: 3 in, 1 out]
          }
        }
        n226 = call <userlib>:"tm_startrecorder_40.vi"("Buffering Mode"=w573, "error in (no error)"=w581, "frames"=w560, "File"=w548, "Handle in"=w582) -> ("error out"=w576:errorcluster, "Handle out"=w574:u32)  [unwired: 5 in]
        n227 = Bundle By Name(cluster=T4 {"frequency"=0.0, "amplitude"=0.0, "offset"=0.0, "phase"=0.0}, "frequency"=w555, "amplitude"=w522, "offset"=w535, "phase"=w536) -> (w551:T4)
        n228 = call "Generate analogue out waveform.vi"("sampling info"=w517, "Reset signal"=TRUE, "error in (no error)"=w516, "Camera start trigger phase"=w532, "Vetl sine"=w550, "Vgalvo sine"=w551) -> ("error out"=w553:errorcluster, "Waveform Graph"=w552:waveform(dbl)[])  [unwired: 4 in]
        n229 = call-poly <vilib>:"DAQmx Write.vi"("task/channels in"=w518, "data"=w552, "error in"=w553) -> ("task out"=w557:refnum<k21>, "error out"=w556:errorcluster)  [unwired: 10 in, 1 out]
        n230 = Create Folder(path (use dialog)=w568) -> (created path=w547:path)  [unwired: 2 in, 2 out]
        n231 = Merge Errors(w556, w576) -> (w575:errorcluster)
        n232 = call <userlib>:"tm_startcapture_40.vi"("error in (no error)"=w575, "Handle in"=w574) -> ("error out"=w559:errorcluster, "Handle out"=w561:u32)  [unwired: 8 in]
        n233 = call <vilib>:"DAQmx Start Task.vi"("task/channels in"=w557, "error in"=w559) -> ("task out"=w546:refnum<k21>, "error out"=w558:errorcluster)  [unwired: 12 in]
        n234 = case shown="No Error" w558 {
          selector: w558 -> [w588 w598]
          tunnel: [w586 w597] -> w565
          tunnel: [w585 w598] -> w564
          tunnel: w560 -> [w587 _]
          tunnel: w561 -> [w584 w597]
          frame No Error {
            n235 = while {
              tunnel: w588 -> [w594]
              tunnel: [w593] -> w585
              tunnel: [w595] -> w586
              tunnel: w587 -> [w596]
              tunnel: w584 -> [w589]
              stop <- w590 stop-if-true
              n236 = Wait (ms)(milliseconds to wait=u32 500) -> ()  [unwired: 1 out]
              n237 = call <userlib>:"tm_getrecorderstatus_40.vi"("error in (no error)"=w594, "Handle"=w589) -> ("error out"=w593:errorcluster, "Count"=w592:i32, "Handle"=w595:u32)  [unwired: 6 in, 1 out]
              n238 = Greater Or Equal?(x=w592, y=w596) -> (x >= y?=w590:bool)
            }
          }
          frame Error {
          }
        }
        n239 = call <userlib>:"tm_stopcapture_40.vi"("error in (no error)"=w564, "Handle in"=w565) -> ("error out"=w562:errorcluster, "Handle out"=w563:u32)  [unwired: 8 in]
        n240 = call <userlib>:"tm_stoprecorder_40.vi"("error in (no error)"=w562, "Handle in"=w563) -> ("error out"=w566:errorcluster, "Handle out"=w567:u32)  [unwired: 8 in]
        n241 = call <userlib>:"tm_unpreparecapture_40.vi"("error in (no error)"=w566, "Handle in"=w567) -> ("error out"=w541:errorcluster, "Handle out"=w544:u32)  [unwired: 8 in]
        n242 = call "from DCIMG to TIFF_sequence.vi"("error in (no error)"=w541, "Where to Store"=w547, "DCIMG Path"=w548) -> ("Error Out"=w540:errorcluster)  [unwired: 7 in, 1 out]
        n243 = call <vilib>:"DAQmx Stop Task.vi"("task/channels in"=w546, "error in"=w541) -> ("task out"=w543:refnum<k21>, "error out"=w542:errorcluster)  [unwired: 12 in]
        n244 = local read "Stop"() -> (w537:bool)
        n245 = Merge Errors(w542, w540) -> (w539:errorcluster)
        n246 = Unbundle By Name(w539) -> ("status"=w545:bool)
        n247 = Or(x=w545, y=w537) -> (x .or. y?=w538:bool)
      }
      n248 = local read "Vgalvo phase 3"() -> (w431:dbl)
      n249 = local read "Vgalvo offset 3"() -> (w430:dbl)
      n250 = local read "Frequency 3"() -> (w432:dbl)
      n251 = local read "Vetl amplitude 3"() -> (w427:dbl)
      n252 = local read "Vetl offset 3"() -> (w429:dbl)
      n253 = local read "Vetl phase 3"() -> (w428:dbl)
      n254 = call <userlib>:"tm_closecamera_40.vi"("error in (no error)"=w460, "Handle in"=w465) -> ("error out"=w464:errorcluster)  [unwired: 9 in]
      n255 = call "MATLAB_find_phase_offset_amplitude_function.vi"("error in (no error)"=w460, "Path"=w461) -> ("error out"=w458:errorcluster, "XY Graph"=w447:cluster{"Array":dbl[], "Array":dbl[]})  [unwired: 7 in, 1 out]
      n256 = call <vilib>:"DAQmx Clear Task.vi"("task in"=w466, "error in"=w460) -> ("error out"=w418:errorcluster)  [unwired: 13 in]
      n257 = Delete(path (use dialog)=w463, entire hierarchy (F)=TRUE, error in=w460) -> (error out=w457:errorcluster)  [unwired: 2 in, 2 out]
      n258 = call <userlib>:"tm_deinitialize_40.vi"("error in (no error)"=w464) -> ("error out"=w459:errorcluster)  [unwired: 10 in]
      n259 = call "0_Control laser.vi"("error in (no error)"=w418, "Laser On/Off"=FALSE ("Layser On/Off")) -> ("error out"=w419:errorcluster)  [unwired: 9 in]
      n260 = Number To Fractional String(number=w432) -> (F-format string=w424:string)  [unwired: 3 in]
      n261 = Number To Fractional String(number=w431) -> (F-format string=w444:string)  [unwired: 3 in]
      n262 = Number To Fractional String(number=w430) -> (F-format string=w442:string)  [unwired: 3 in]
      n263 = Number To Fractional String(number=w427) -> (F-format string=w440:string)  [unwired: 3 in]
      n264 = Number To Fractional String(number=w429) -> (F-format string=w438:string)  [unwired: 3 in]
      n265 = Number To Fractional String(number=w428) -> (F-format string=w436:string)  [unwired: 3 in]
      n266 = Merge Errors(w419, w459, w458, w457) -> (w446:errorcluster)
      n267 = Concatenate Strings(w433, ": Frequency=", w424, "  VgP=", w444, "  O=", w442, "  VeA=", w440, "  O=", w438, "  P=", w436, "\r\n") -> (w435:string)
    }
  }
  "error out" <- w3
  "XY Graph" <- w16
  n268 = Path To String(path=w12) -> (string=w15:string)
  n269 = Concatenate Strings(w15, "\\log.txt") -> (w13:string)
  n270 = String To Path(string=w13) -> (path=w11:path)
  n271 = Open/Create/Replace File(file path (use dialog)=w11, operation (0:open)=T3."open or create") -> (refnum out=w9:refnum<file>)  [unwired: 4 in, 2 out]
  n272 = Set File Position(offset (in bytes) (0)=i64 0, refnum=w9, from (0:start)=enum16{"start", "end", "current"}."end") -> (refnum out=w6:refnum<file>)  [unwired: 1 in, 1 out]
  n273 = call <vilib>:"Simple Error Handler.vi"("error in (no error)"=w3) -> ()  [unwired: 4 in, 5 out]
  n274 = Write to Text File(file (use dialog)=w6, text=w5, error in=w3) -> (refnum out=w4:refnum<file>, error out=w2:errorcluster)  [unwired: 1 in, 1 out]
  n275 = Close File(refnum=w4, error in=w2) -> ()  [unwired: 2 out]
